vi "Remove Pending Transfer.vi"(8 "error in":errorcluster, 10 "SDO Transfer":refnum<class "SDO Transfer.lvclass">, 11 "Pending Transfers":refnum<data-value>) -> (0 "error out":errorcluster, 2 "Removed SDO Transfer":refnum<class "SDO Transfer.lvclass">)   [LabVIEW 2020, in "CANopen.lvlib" / "SDO Manager.lvlib" / "SDO Manager.lvclass"]
uses:
  SDO Manager.lvclass
  SDO Transfer/SDO Transfer.lvclass
  Response Matcher/IResponse/IMatch Response.lvclass
  SDO Transfer/SDO Transfer.lvclass/SDO Transfer.ctl
  SDO Manager.lvclass/SDO Manager.ctl
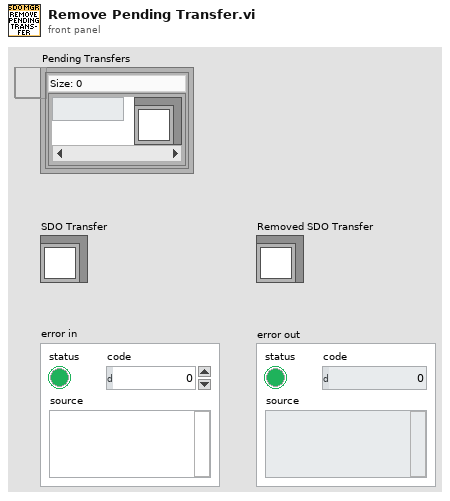
[diagram p1: front panel]
types:
  T1 = map{string, refnum<class "IMatch Response.lvclass">}
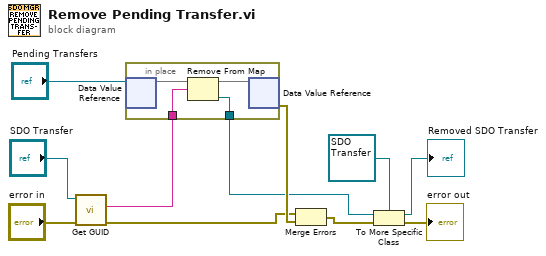
[diagram p0: block diagram]
diagram:
  n1 = call "Get GUID.vi"("error in"="error in", "SDO Transfer in"="SDO Transfer") -> ("error out"=w7:errorcluster, "GUID"=w5:string)  [unwired: 7 in, 1 out]
  n2 = in-place {
    in-place-border: [w13] -> w2
    in-place-border: w5 -> [w12]
    n3 = in-place-dvr #1("Pending Transfers") -> (w15:T1)  [unwired: 1 out]
    n4 = Remove From Map(10:w12, 11:w15) -> (1:w13:refnum<class "IMatch Response.lvclass">, 3:w14:T1)  [unwired: 1 out]
    n5 = in-place-dvr #1(w14) -> (w8:errorcluster)  [unwired: 1 out]
  }
  n6 = Merge Errors(w7, w8) -> (w10:errorcluster)
  n7 = To More Specific Class(target class=refnum<class "SDO Transfer.lvclass"> refnum ("CANopen.lvlib:SDO Manager.lvlib:SDO Transfer"), reference=w2, error in=w10) -> (specific class reference=→"Removed SDO Transfer":refnum<class "SDO Transfer.lvclass">, error out=→"error out":errorcluster)
